vi "HEX2文本.vi"(10 "读内部参数":string[](array[string])) -> (2 "内部参数(文本)":string[](array[string]))   [LabVIEW 2015]
panel:
  out "反向功率dBm":dbl
  out "正向功率dBm":dbl
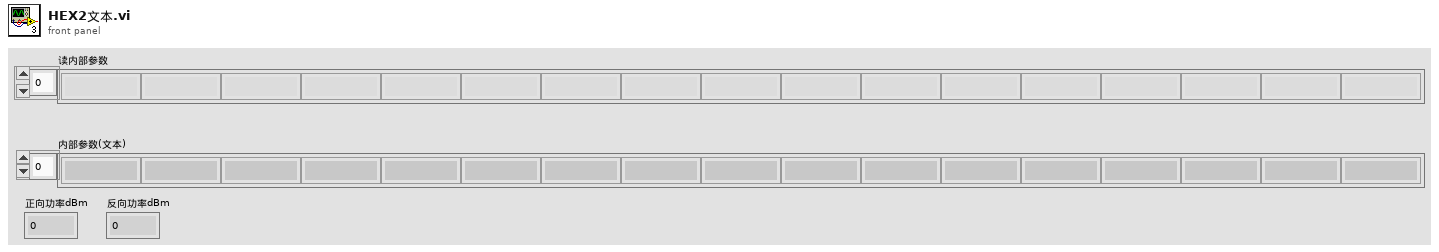
[diagram p1: front panel]
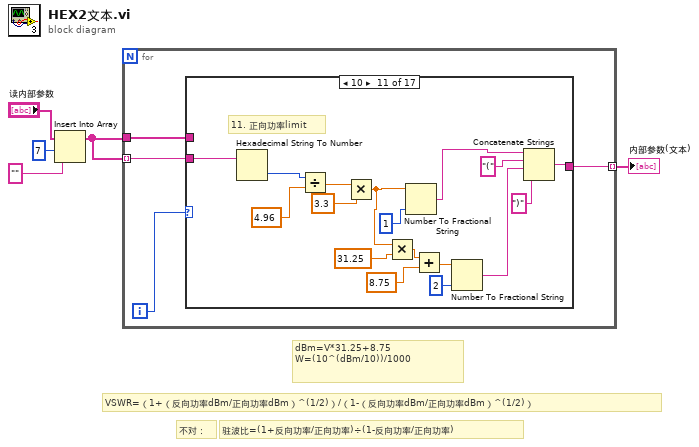
[diagram p0: block diagram]
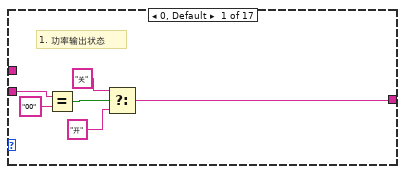
[diagram p2: hidden frame]
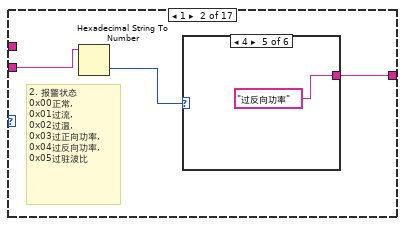
[diagram p3: hidden frame]
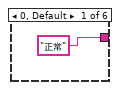
[diagram p4: hidden frame]
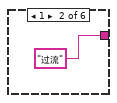
[diagram p5: hidden frame]
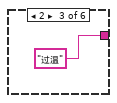
[diagram p6: hidden frame]
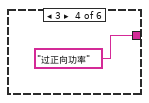
[diagram p7: hidden frame]
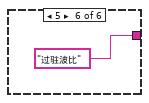
[diagram p8: hidden frame]
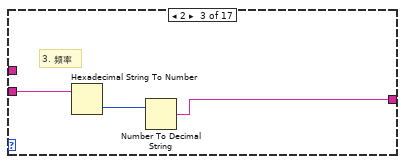
[diagram p9: hidden frame]
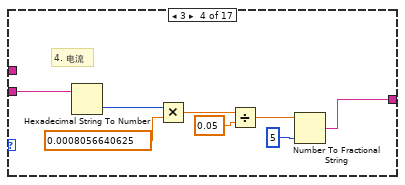
[diagram p10: hidden frame]
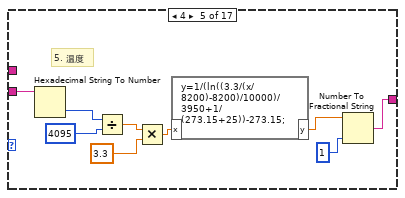
[diagram p11: hidden frame]
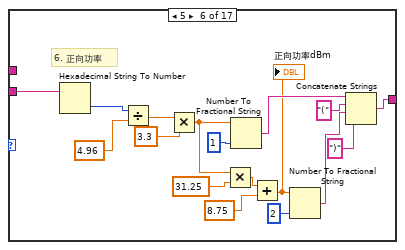
[diagram p12: hidden frame]
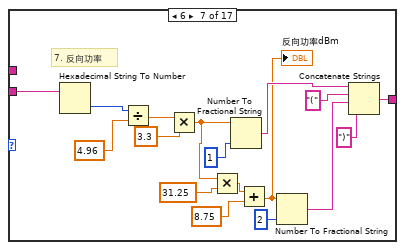
[diagram p13: hidden frame]
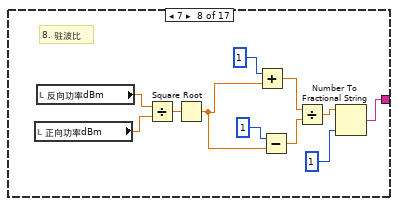
[diagram p14: hidden frame]
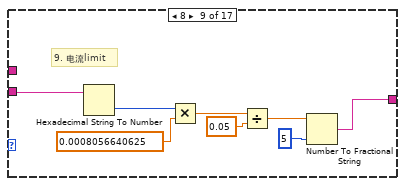
[diagram p15: hidden frame]
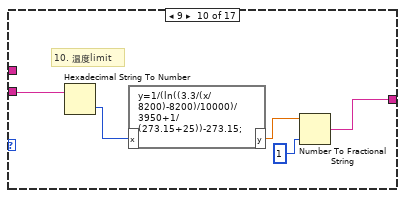
[diagram p16: hidden frame]
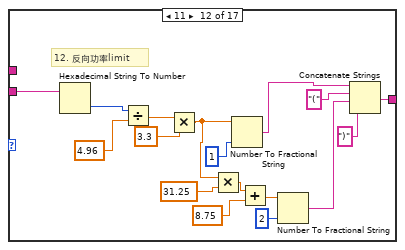
[diagram p17: hidden frame]
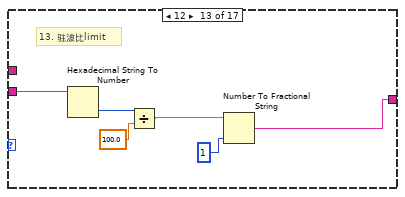
[diagram p18: hidden frame]
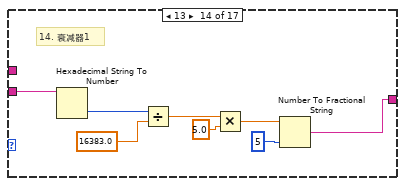
[diagram p19: hidden frame]
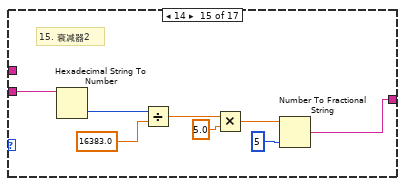
[diagram p20: hidden frame]
diagram:
  # "不对："
  # "驻波比=(1+反向功率/正向功率)÷(1-反向功率/正向功率)"
  # "VSWR=（1+（反向功率dBm/正向功率dBm）^(1/2)）/（1-（反向功率dBm/正向功率dBm）^(1/2)）"
  # "dBm=V*31.25+8.75\nW=(10^(dBm/10))/1000"
  n1 = Insert Into Array(array="读内部参数", index=7 ("索引"), new element="" ("新元素/子数组")) -> (w1:string[])
  n2 = for {
    tunnel: w1 -> [w8] mode=indexing
    tunnel: [w7] -> w5 mode=indexing
    tunnel: w1 -> [w6]
    i -> [w9]
    n3 = case shown="10" w9 {
      tunnel: w8 -> [w15 w18 w27 w35 w44 w61 w78 _ w91 w99 w119 w136 w142 w144 w152 w160 w168]
      tunnel: [w10 w16 w25 w28 w42 w53 w65 w84 w90 w98 w104 w121 w137 w143 w151 w159 w167] -> w7
      tunnel: w6 -> [_ _ _ _ _ _ _ _ _ _ _ _ _ _ _ _ _]
      frame 0, Default {
        # "1.\t功率输出状态"
        n4 = Equal?(x=w15, y="00") -> (x = y?=w13:bool)
        n5 = Select(t="关" ("y"), s=w13, f="开" ("y")) -> (s? t:f=w10:string)
      }
      frame 1 {
        # "2.\t报警状态\n0x00正常,\n0x01过流,\n0x02过温,\n0x03过正向功率,\n0x04过反向功率,\n0x05过驻波比"
        n6 = Hexadecimal String To Number(string=w18) -> (number=w17:u32)  [unwired: 2 in, 1 out]
        n7 = case shown="4" w17 {
          tunnel: ["正常" "过流" "过温" "过正向功率" "过反向功率" "过驻波比"] -> w16
          frame 0, Default {
          }
          frame 1 {
          }
          frame 2 {
          }
          frame 3 {
          }
          frame 4 {
          }
          frame 5 {
          }
        }
      }
      frame 2 {
        # "3.\t频率"
        n8 = Hexadecimal String To Number(string=w27) -> (number=w26:u32)  [unwired: 2 in, 1 out]
        n9 = Number To Decimal String(number=w26) -> (decimal integer string=w25:string)  [unwired: 1 in]
      }
      frame 3 {
        # "4.\t电流"
        n10 = Hexadecimal String To Number(string=w35) -> (number=w29:u32)  [unwired: 2 in, 1 out]
        n11 = Multiply(x=w29, y=0.0008056640625) -> (x*y=w31:dbl)
        n12 = Divide(x=w31, y=0.05) -> (x/y=w33:dbl)
        n13 = Number To Fractional String(number=w33, precision (6)=i16 5 ("精度(6)")) -> (F-format string=w28:string)  [unwired: 2 in]
      }
      frame 4 {
        # "5.\t温度"
        n14 = Hexadecimal String To Number(string=w44) -> (number=w37:u32)  [unwired: 2 in, 1 out]
        n15 = Divide(x=w37, y=u16 4095) -> (x/y=w39:dbl)
        n16 = Multiply(x=w39, y=3.3) -> (x*y=w36:dbl)
        n17 = formula code="y=1/(ln((3.3/(x/8200)-8200)/10000)/3950+1/(273.15+25))-273.15;"("x"=w36) -> ("y"=w41:dbl)
        n18 = Number To Fractional String(number=w41, precision (6)=i16 1 ("精度(6)")) -> (F-format string=w42:string)  [unwired: 2 in]
      }
      frame 5 {
        # "6.\t正向功率"
        n19 = Hexadecimal String To Number(string=w61) -> (number=w59:u32)  [unwired: 2 in, 1 out]
        n20 = Divide(x=w59, y=4.96) -> (x/y=w57:dbl)
        n21 = Multiply(x=w57, y=3.3) -> (x*y=w52:dbl)
        n22 = Multiply(x=w52, y=31.25) -> (x*y=w50:dbl)
        n23 = Number To Fractional String(number=w52, precision (6)=i16 1 ("精度(6)")) -> (F-format string=w55:string)  [unwired: 2 in]
        n24 = Add(x=w50, y=8.75) -> (x+y=w47:dbl)
        "正向功率dBm" <- w47
        n25 = Number To Fractional String(number=w47, precision (6)=i16 2 ("精度(6)")) -> (F-format string=w45:string)  [unwired: 2 in]
        n26 = Concatenate Strings(w55, "(" ("字符串"), w45, ")" ("字符串")) -> (w53:string)
      }
      frame 6 {
        # "7.\t反向功率"
        n27 = Hexadecimal String To Number(string=w78) -> (number=w76:u32)  [unwired: 2 in, 1 out]
        n28 = Divide(x=w76, y=4.96) -> (x/y=w74:dbl)
        n29 = Multiply(x=w74, y=3.3) -> (x*y=w68:dbl)
        n30 = Multiply(x=w68, y=31.25) -> (x*y=w71:dbl)
        n31 = Number To Fractional String(number=w68, precision (6)=i16 1 ("精度(6)")) -> (F-format string=w64:string)  [unwired: 2 in]
        n32 = Add(x=w71, y=8.75) -> (x+y=w62:dbl)
        "反向功率dBm" <- w62
        n33 = Number To Fractional String(number=w62, precision (6)=i16 2 ("精度(6)")) -> (F-format string=w63:string)  [unwired: 2 in]
        n34 = Concatenate Strings(w64, "(" ("字符串"), w63, ")" ("字符串")) -> (w65:string)
      }
      frame 7 {
        # "8.\t驻波比"
        n35 = local read "正向功率dBm"() -> (w80:dbl)
        n36 = local read "反向功率dBm"() -> (w81:dbl)
        n37 = Divide(x=w81, y=w80) -> (x/y=w82:dbl)
        n38 = Square Root(x=w82) -> (sqrt(x)=w79:dbl)
        n39 = Add(x=1, y=w79) -> (x+y=w87:dbl)
        n40 = Subtract(x=1, y=w79) -> (x-y=w86:dbl)
        n41 = Divide(x=w87, y=w86) -> (x/y=w85:dbl)
        n42 = Number To Fractional String(number=w85, precision (6)=i16 1 ("精度(6)")) -> (F-format string=w84:string)  [unwired: 2 in]
      }
      frame 8 {
        # "9.\t电流limit"
        n43 = Hexadecimal String To Number(string=w91) -> (number=w92:u32)  [unwired: 2 in, 1 out]
        n44 = Multiply(x=w92, y=0.0008056640625) -> (x*y=w94:dbl)
        n45 = Divide(x=w94, y=0.05) -> (x/y=w96:dbl)
        n46 = Number To Fractional String(number=w96, precision (6)=i16 5 ("精度(6)")) -> (F-format string=w90:string)  [unwired: 2 in]
      }
      frame 9 {
        # "10.\t温度limit"
        n47 = Hexadecimal String To Number(string=w99) -> (number=w101:u32)  [unwired: 2 in, 1 out]
        n48 = formula code="y=1/(ln((3.3/(x/8200)-8200)/10000)/3950+1/(273.15+25))-273.15;"("x"=w101) -> ("y"=w100:dbl)
        n49 = Number To Fractional String(number=w100, precision (6)=i16 1 ("精度(6)")) -> (F-format string=w98:string)  [unwired: 2 in]
      }
      frame 10 {
        # "11.\t正向功率limit"
        n50 = Hexadecimal String To Number(string=w119) -> (number=w118:u32)  [unwired: 2 in, 1 out]
        n51 = Divide(x=w118, y=4.96) -> (x/y=w116:dbl)
        n52 = Multiply(x=w116, y=3.3) -> (x*y=w105:dbl)
        n53 = Multiply(x=w105, y=31.25) -> (x*y=w112:dbl)
        n54 = Number To Fractional String(number=w105, precision (6)=i16 1 ("精度(6)")) -> (F-format string=w107:string)  [unwired: 2 in]
        n55 = Add(x=w112, y=8.75) -> (x+y=w103:dbl)
        n56 = Number To Fractional String(number=w103, precision (6)=i16 2 ("精度(6)")) -> (F-format string=w106:string)  [unwired: 2 in]
        n57 = Concatenate Strings(w107, "(" ("字符串"), w106, ")" ("字符串")) -> (w104:string)
      }
      frame 11 {
        # "12.\t反向功率limit"
        n58 = Hexadecimal String To Number(string=w136) -> (number=w135:u32)  [unwired: 2 in, 1 out]
        n59 = Divide(x=w135, y=4.96) -> (x/y=w133:dbl)
        n60 = Multiply(x=w133, y=3.3) -> (x*y=w122:dbl)
        n61 = Multiply(x=w122, y=31.25) -> (x*y=w129:dbl)
        n62 = Number To Fractional String(number=w122, precision (6)=i16 1 ("精度(6)")) -> (F-format string=w124:string)  [unwired: 2 in]
        n63 = Add(x=w129, y=8.75) -> (x+y=w120:dbl)
        n64 = Number To Fractional String(number=w120, precision (6)=i16 2 ("精度(6)")) -> (F-format string=w123:string)  [unwired: 2 in]
        n65 = Concatenate Strings(w124, "(" ("字符串"), w123, ")" ("字符串")) -> (w121:string)
      }
      frame 12 {
        # "13.\t驻波比limit"
        n66 = Hexadecimal String To Number(string=w142) -> (number=w141:u32)  [unwired: 2 in, 1 out]
        n67 = Divide(x=w141, y=100.0) -> (x/y=w138:dbl)
        n68 = Number To Fractional String(number=w138, precision (6)=i16 1 ("精度(6)")) -> (F-format string=w137:string)  [unwired: 2 in]
      }
      frame 13 {
        # "14.\t衰减器1"
        n69 = Hexadecimal String To Number(string=w144) -> (number=w145:u32)  [unwired: 2 in, 1 out]
        n70 = Divide(x=w145, y=16383.0) -> (x/y=w147:dbl)
        n71 = Multiply(x=w147, y=5.0) -> (x*y=w149:dbl)
        n72 = Number To Fractional String(number=w149, precision (6)=i16 5 ("精度(6)")) -> (F-format string=w143:string)  [unwired: 2 in]
      }
      frame 14 {
        # "15.\t衰减器2"
        n73 = Hexadecimal String To Number(string=w152) -> (number=w153:u32)  [unwired: 2 in, 1 out]
        n74 = Divide(x=w153, y=16383.0) -> (x/y=w155:dbl)
        n75 = Multiply(x=w155, y=5.0) -> (x*y=w157:dbl)
        n76 = Number To Fractional String(number=w157, precision (6)=i16 5 ("精度(6)")) -> (F-format string=w151:string)  [unwired: 2 in]
      }
      frame 15 {
        # "16.\t偏置1"
        n77 = Hexadecimal String To Number(string=w160) -> (number=w161:u32)  [unwired: 2 in, 1 out]
        n78 = Divide(x=w161, y=16383.0) -> (x/y=w163:dbl)
        n79 = Multiply(x=w163, y=5.0) -> (x*y=w165:dbl)
        n80 = Number To Fractional String(number=w165, precision (6)=i16 5 ("精度(6)")) -> (F-format string=w159:string)  [unwired: 2 in]
      }
      frame 16 {
        # "17.\t偏置2"
        n81 = Hexadecimal String To Number(string=w168) -> (number=w169:u32)  [unwired: 2 in, 1 out]
        n82 = Divide(x=w169, y=16383.0) -> (x/y=w171:dbl)
        n83 = Multiply(x=w171, y=5.0) -> (x*y=w173:dbl)
        n84 = Number To Fractional String(number=w173, precision (6)=i16 5 ("精度(6)")) -> (F-format string=w167:string)  [unwired: 2 in]
      }
    }
  }
  "内部参数(文本)" <- w5
